vi "CRYOpen All.vi"   [LabVIEW 2013]
uses:
  CRYSystem/Typedef Control/CRYData Cluster.ctl
  CRYSystem/Typedef Control/CRYWaveform Cluster.ctl
  Global/CRYCurve Library Global.vi
panel:
  # "Open All Data(Curves, Values,Results, Waveforms)"
types:
  T1 = cluster{"pattern label":string, "pattern":string}
  T2 = cluster{"pattern label":string, "pattern":string}[]
  T3 = enum16{"Left Button", "Center Button", "Right Button", "Window Close"}
  T4 = enum16{"OK", "Yes", "YesNo", "YesNoCancel", "ReplaceAppend"}
  T5 = cluster{"Color":u32, "Interpolation":u8, "Point Style":u8, "Line Style":u8, "Point Color":u32, "Line Width":u8, "Bar Plot Style":u8, "Fill To":i16}
  T6 = typedef "CRYData Cluster.ctl" = cluster{"Name":string, "Curve":cluster{"x":dbl, "y":dbl, "z":dbl}[], "X data":u16, "Y data":u16, "Z data":u16, "X axis":u16, "Y axis":u16, "Z axis":u16, "X unit":string, "Y unit":string, "Z unit":string, "X dB ref":dbl, "Y dB ref":dbl, "Z dB ref":dbl, "single val":bool, "protected":bool, "display X":bool, "display Y":bool, "display Z":bool, "Test Info":string, "Step No.":i32, "Plot Settings":cluster{"Color":u32, "Interpolation":u8, "Point Style":u8, "Line Style":u8, "Point Color":u32, "Line Width":u8, "Bar Plot Style":u8, "Fill To":i16}, "AutoProtect":bool}
  T7 = typedef "CRYResult Cluster.ctl" = cluster{"Name":string, "Margin":dbl, "unit":string, "Verdict":bool, "Limit":string, "Max/Min":string, "protected":bool, "Step No.":i32, "Test Info":string, "AutoProtect":bool}
  T8 = typedef "CRYWaveform Cluster.ctl" = cluster{"Waveform":cluster{"X0":dbl, "dX":dbl, "Y":sgl[]}, "X data":u16, "Y data":u16, "Y axis":u16, "X unit":string, "Y unit":string, "Y dB ref":dbl, "display Y":bool, "display X":bool, "Overload?":bool, "Test Info":string, "Step No.":i32, "Name":string, "protected":bool, "Sqc history":string[], "Signal Channel ID":i32, "Plot Settings":cluster{"Color":u32, "Interpolation":u8, "Point Style":u8, "Line Style":u8, "Point Color":u32, "Line Width":u8, "Bar Plot Style":u8, "Fill To":i16}, "AutoProtect":bool}
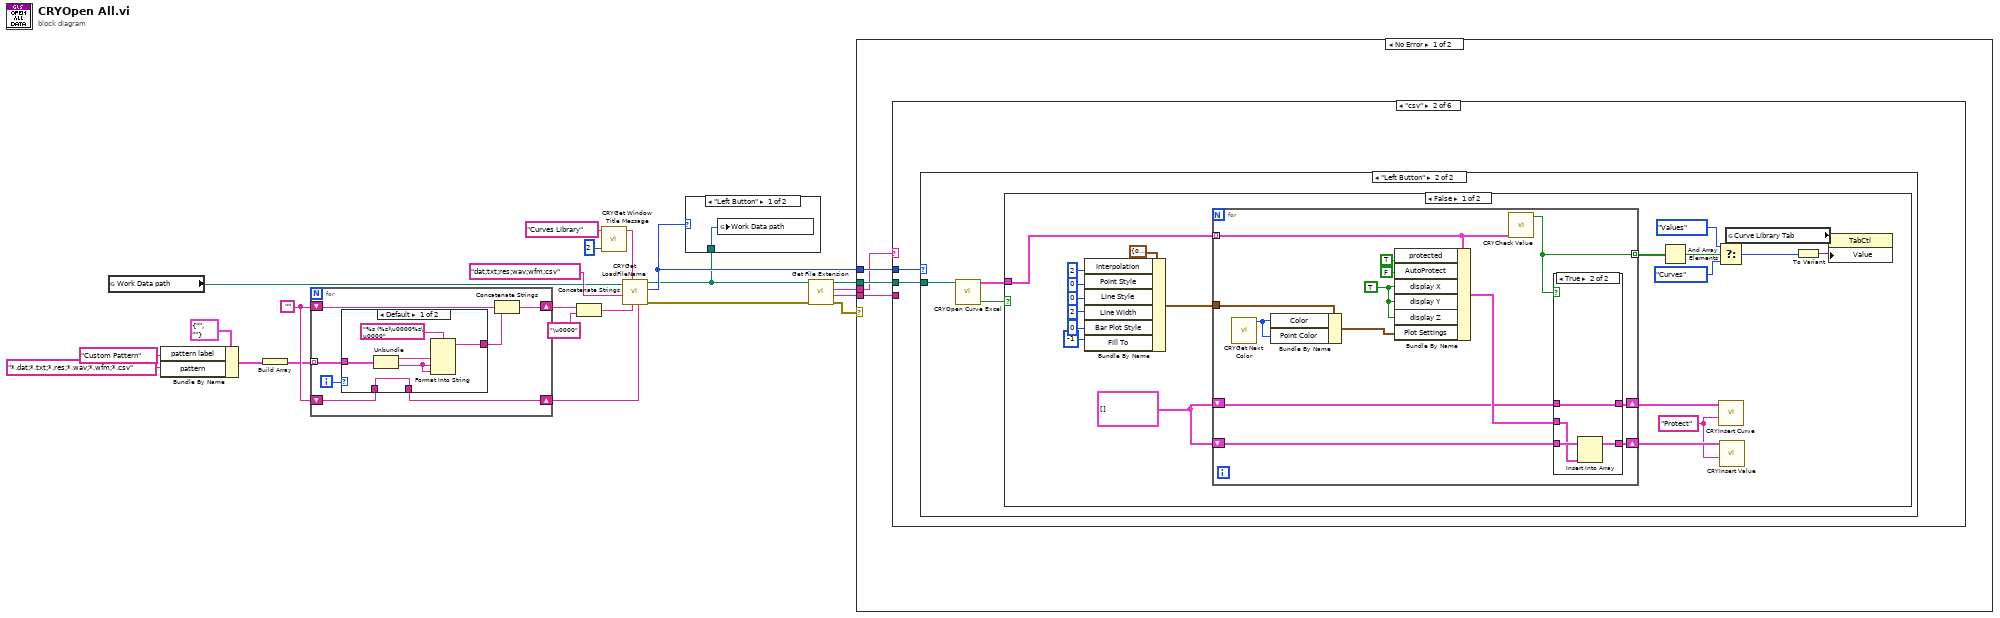
[diagram p0: block diagram]
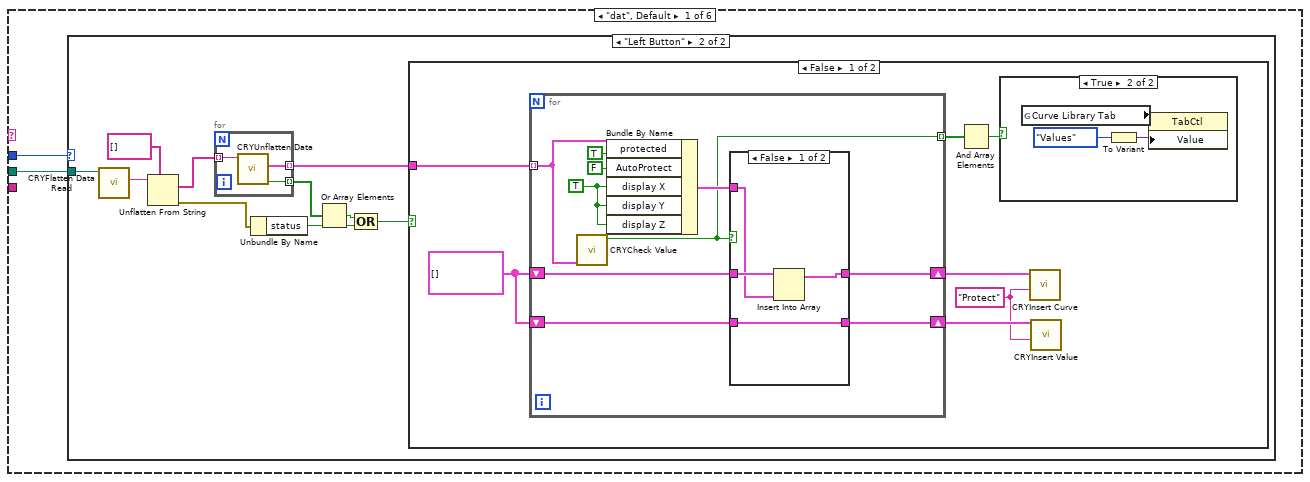
[diagram p3: hidden frame]
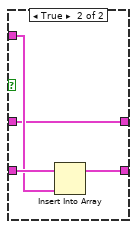
[diagram p6: hidden frame]
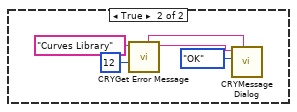
[diagram p7: hidden frame]
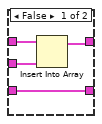
[diagram p9: hidden frame]
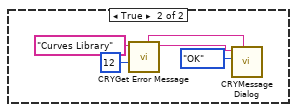
[diagram p10: hidden frame]
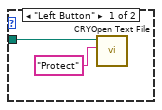
[diagram p12: hidden frame]
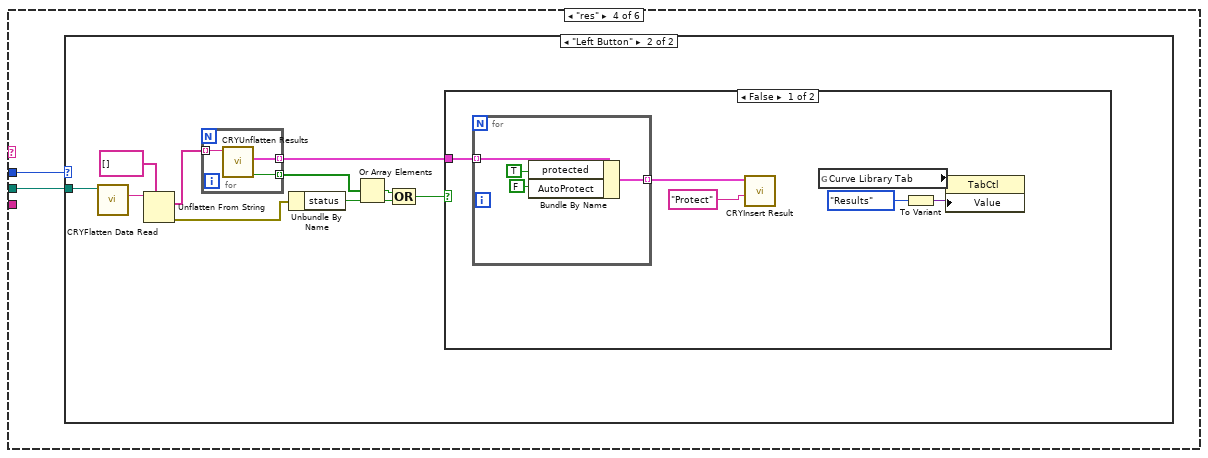
[diagram p13: hidden frame]
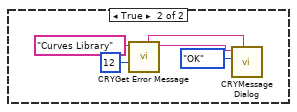
[diagram p15: hidden frame]
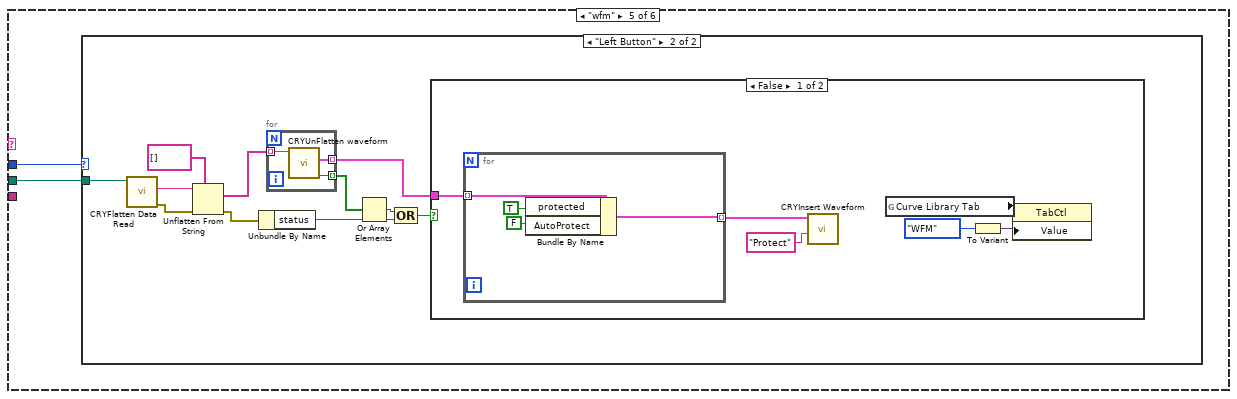
[diagram p16: hidden frame]
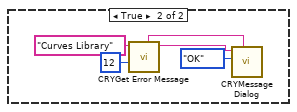
[diagram p18: hidden frame]
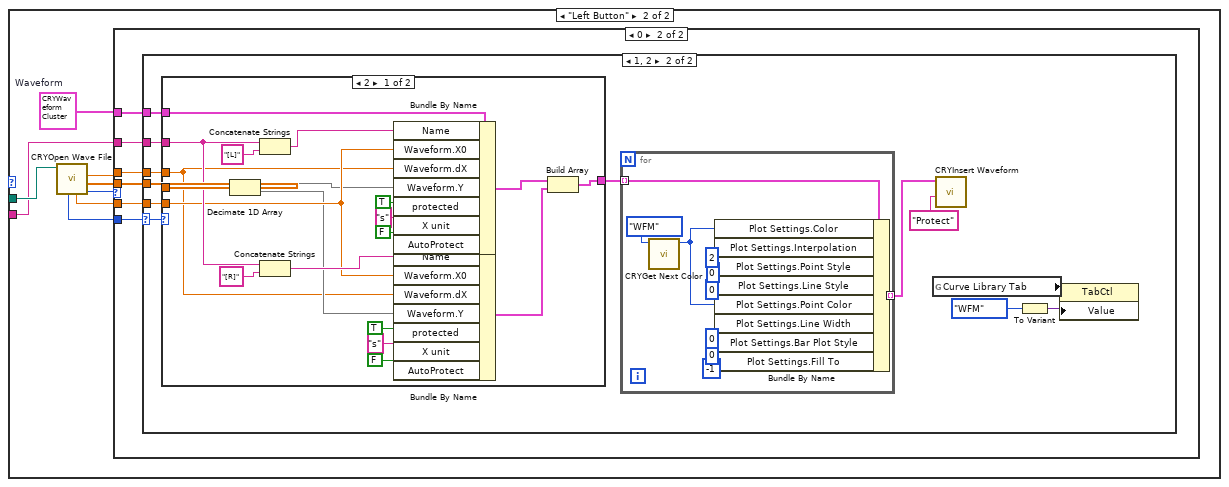
[diagram p20: hidden frame]
diagram:
  w14 = ""
  n1 = global read "CRYCurve Library Global.vi" "Work Data path"() -> (w3:path)
  n2 = Bundle By Name(cluster=T1 {"pattern label"="", "pattern"=""} ("File Types"), "pattern label"="Custom Pattern" ("pattern (all files)"), "pattern"="*.dat;*.txt;*.res;*.wav;*.wfm;*.csv" ("pattern (all files)")) -> (w5:T1)
  n3 = Build Array(w5) -> (w13:T2)
  n4 = for {
    tunnel: w13 -> [w29] mode=indexing
    shift-right: [w28] -> w16
    shift-left: w14 -> [w27]
    shift-right: [w24] -> w12
    shift-left: w14 -> [w23]
    i -> [w26]
    n5 = case shown="Default" w26 {
      tunnel: w29 -> [w35 w40]
      tunnel: [w31 w37] -> w25
      tunnel: [w30 w36] -> w24
      tunnel: w23 -> [w30 _]
      frame Default {
        n6 = Unbundle(w35) -> ("pattern label"=w34:string, "pattern"=w32:string)
        n7 = Format Into String(format string="%s (%s)\u0000%s\u0000", w34, w32, w32) -> (resulting string=w31:string)  [unwired: 2 in, 1 out]
      }
      frame 0 {
        n8 = Unbundle(w40) -> ("pattern label"=w36:string, "pattern"=w38:string)
        n9 = Format Into String(format string="%s)\u0000%s\u0000", w38, w38) -> (resulting string=w37:string)  [unwired: 2 in, 1 out]
      }
    }
    n10 = Concatenate Strings(w27, w25) -> (w28:string)
  }
  n11 = Concatenate Strings(w16, "\u0000" ("format string")) -> (w11:string)
  n12 = call "CRYGet Window Title Message.vi"("No"=2 ("Error No"), "Kind"="Curves Library") -> ("Multibyte String"=w17:string)  [unwired: 4 in, 5 out]
  n13 = call "CRYGet LoadFileName.vi"("pattern label"=w12, "pattern (all files)"=w11, "TitleName"=w17, "Category Name"="dat;txt;res;wav;wfm;csv" ("pattern (all files)"), "Start path"=w3) -> ("error out"=w21:errorcluster, "Which Button?"=w2:T3, "Path"=w1:path)  [unwired: 3 in, 1 out]
  n14 = case shown="\"Left Button\"" w2 {
    tunnel: w1 -> [w41 _]
    frame "Left Button" {
      n15 = global write "CRYCurve Library Global.vi" "Work Data path"(w41) -> ()
    }
    frame "Center Button", Default {
    }
  }
  n16 = call <vilib>:"Get File Extension.vi"("error in (no error)"=w21, "file"=w1) -> ("error out"=w9:errorcluster, "filename without extension"=w20:string, "lowercase file extension"=w19:string, "dup file"=w22:path)  [unwired: 6 out]
  n17 = case shown="No Error" w9 {
    tunnel: w2 -> [w45 _]
    tunnel: w22 -> [w44 _]
    tunnel: w20 -> [w43 _]
    tunnel: w19 -> [w42 _]
    frame No Error {
      n18 = case shown="\"csv\"" w42 {
        tunnel: w45 -> [w47 w95 w146 w150 w180 w212]
        tunnel: w44 -> [w46 w94 w145 w149 w179 w211]
        tunnel: w43 -> [_ _ _ _ _ w210]
        frame "dat", Default {
          n19 = case shown="\"Left Button\"" w47 {
            tunnel: w46 -> [_ w57]
            frame "Center Button", Default {
            }
            frame "Left Button" {
              n20 = call "CRYFlatten Data Read.vi"("Path In"=w57) -> ("Flatten Data Out"=w56:string)  [unwired: 1 in, 7 out]
              n21 = Unflatten From String(type=string[] [], binary string=w56) -> (value=w54:string[], error out=w50:errorcluster)  [unwired: 1 in, 3 out]
              n22 = for {
                tunnel: w54 -> [w60] mode=indexing
                tunnel: [w59] -> w53 mode=indexing
                tunnel: [w58] -> w48 mode=indexing
                n23 = call "CRYUnflatten Data.vi"("Unflatten data"=w60) -> ("Error?"=w58:bool, "Datum"=w59:T6)  [unwired: 8 in, 1 out]
              }
              n24 = Unbundle By Name(w50) -> ("status"=w51:bool)
              n25 = Or Array Elements(Boolean array=w48) -> (logical OR=w52:bool)
              n26 = Compound Arithmetic op=OR(w52, w51) -> (w49:bool)
              n27 = case shown="False" w49 {
                tunnel: w53 -> [w65 _]
                frame False {
                  w61 = "Protect" ("sOption")
                  w64 = T6[] []
                  n28 = for {
                    tunnel: w65 -> [w79] mode=indexing
                    tunnel: [w78] -> w67 mode=indexing
                    shift-right: [w71] -> w63
                    shift-left: w64 -> [w74]
                    shift-right: [w72] -> w62
                    shift-left: w64 -> [w73]
                    w75 = TRUE ("display X")
                    n29 = call "CRYCheck Value.vi"("Data"=w79) -> ("Single?"=w78:bool)  [unwired: 2 in, 8 out]
                    n30 = Bundle By Name(cluster=w79, "protected"=TRUE, "AutoProtect"=FALSE, "display X"=w75, "display Y"=w75, "display Z"=w75) -> (w80:T6)
                    n31 = case shown="False" w78 {
                      tunnel: w80 -> [w83 w87]
                      tunnel: w74 -> [w84 w85]
                      tunnel: w73 -> [w81 w88]
                      tunnel: [w81 w86] -> w72
                      tunnel: [w82 w85] -> w71
                      frame False {
                        n32 = Insert Into Array(array=w84, new element=w83) -> (w82:T6[])  [unwired: 1 in]
                      }
                      frame True {
                        n33 = Insert Into Array(array=w88, new element=w87) -> (w86:T6[])  [unwired: 1 in]
                      }
                    }
                  }
                  n34 = And Array Elements(Boolean array=w67) -> (logical AND=w66:bool)
                  n35 = case shown="True" w66 {
                    frame False {
                    }
                    frame True {
                      n36 = global read "CRYCurve Library Global.vi" "Curve Library Tab"() -> (w70:refnum<vi>)
                      n37 = To Variant(anything=enum32{"Curves", "Values", "Results", "WFM"}."Values" ("Value")) -> (Variant=w68:variant)
                      n38 = property class="TabCtl"(reference=w70, "Value"=w68) -> ()  [unwired: 1 in, 2 out]
                    }
                  }
                  n39 = call "CRYInsert Curve.vi"("sOption"=w61, "Curve"=w63) -> ()  [unwired: 2 in, 8 out]
                  n40 = call "CRYInsert Value.vi"("sOption"=w61, "Value"=w62) -> ()  [unwired: 2 in, 8 out]
                }
                frame True {
                  n41 = call "CRYGet Error Message.vi"("Error No"=12, "Kind"="Curves Library") -> ("Message"=w90:string, "Window Title"=w89:string)  [unwired: 4 in, 4 out]
                  n42 = call "CRYMessage Dialog.vi"("Window Title"=w89, "YesNoCancel"=T4."OK", "Message Content"=w90) -> ()  [unwired: 7 in, 2 out]
                }
              }
            }
          }
        }
        frame "csv" {
          n43 = case shown="\"Left Button\"" w95 {
            tunnel: w94 -> [_ w98]
            frame "Center Button", Default {
            }
            frame "Left Button" {
              n44 = call "CRYOpen Curve Excel .vi"("file path (dialog if empty)"=w98) -> ("Return"=w96:bool, "Data"=w97:T6[])  [unwired: 9 in]
              n45 = case shown="False" w96 {
                tunnel: w97 -> [w117 _]
                frame False {
                  w113 = "Protect" ("sOption")
                  w116 = T6[] []
                  n46 = Bundle By Name(cluster=T5 {"Color"=0, "Interpolation"=0, "Point Style"=0, "Line Style"=0, "Point Color"=0, "Line Width"=0, "Bar Plot Style"=0, "Fill To"=0} ("Plot Settings"), "Interpolation"=u8 2 ("Plot Settings.Interpolation"), "Point Style"=u8 0 ("Plot Settings.Point Style"), "Line Style"=u8 0 ("Plot Settings.Line Style"), "Line Width"=u8 2 ("Plot Settings.Line Width"), "Bar Plot Style"=u8 0 ("Plot Settings.Bar Plot Style"), "Fill To"=i16 -1 ("Plot Settings.Fill To")) -> (w99:T5)
                  n47 = for {
                    tunnel: w117 -> [w122] mode=indexing
                    tunnel: [w130] -> w118 mode=indexing
                    shift-right: [w123] -> w115
                    shift-left: w116 -> [w126]
                    shift-right: [w124] -> w114
                    shift-left: w116 -> [w125]
                    tunnel: w99 -> [w120]
                    w127 = TRUE ("display X")
                    n48 = call "CRYGet Next Color.vi"() -> ("Color"=w121:u32)  [unwired: 1 in, 10 out]
                    n49 = Bundle By Name(cluster=w120, "Color"=w121, "Point Color"=w121) -> (w119:T5)
                    n50 = Bundle By Name(cluster=w122, "protected"=TRUE, "AutoProtect"=FALSE, "display X"=w127, "display Y"=w127, "display Z"=w127, "Plot Settings"=w119) -> (w131:T6)
                    n51 = call "CRYCheck Value.vi"("Data"=w122) -> ("Single?"=w130:bool)  [unwired: 2 in, 8 out]
                    n52 = case shown="True" w130 {
                      tunnel: w131 -> [w134 w138]
                      tunnel: w126 -> [w135 w136]
                      tunnel: w125 -> [w132 w139]
                      tunnel: [w132 w137] -> w124
                      tunnel: [w133 w136] -> w123
                      frame False {
                        n53 = Insert Into Array(array=w135, new element=w134) -> (w133:T6[])  [unwired: 1 in]
                      }
                      frame True {
                        n54 = Insert Into Array(array=w139, new element=w138) -> (w137:T6[])  [unwired: 1 in]
                      }
                    }
                  }
                  n55 = And Array Elements(Boolean array=w118) -> (logical AND=w110:bool)
                  n56 = Select(t=enum32{"Curves", "Values", "Results", "WFM"}."Values" ("Value"), s=w110, f=enum32{"Curves", "Values", "Results", "WFM"}."Curves" ("Value")) -> (s? t:f=w107:enum32{"Curves", "Values", "Results", "WFM"})
                  n57 = call "CRYInsert Curve.vi"("sOption"=w113, "Curve"=w115) -> ()  [unwired: 2 in, 8 out]
                  n58 = call "CRYInsert Value.vi"("sOption"=w113, "Value"=w114) -> ()  [unwired: 2 in, 8 out]
                  n59 = global read "CRYCurve Library Global.vi" "Curve Library Tab"() -> (w112:refnum<vi>)
                  n60 = To Variant(anything=w107) -> (Variant=w111:variant)
                  n61 = property class="TabCtl"(reference=w112, "Value"=w111) -> ()  [unwired: 1 in, 2 out]
                }
                frame True {
                  n62 = call "CRYGet Error Message.vi"("Error No"=12, "Kind"="Curves Library") -> ("Message"=w141:string, "Window Title"=w140:string)  [unwired: 4 in, 4 out]
                  n63 = call "CRYMessage Dialog.vi"("Window Title"=w140, "YesNoCancel"=T4."OK", "Message Content"=w141) -> ()  [unwired: 7 in, 2 out]
                }
              }
            }
          }
        }
        frame "txt" {
          n64 = case shown="\"Center Button\", Default" w146 {
            tunnel: w145 -> [w148 _]
            frame "Left Button" {
              n65 = call "CRYOpen Text File.vi"("sOption"="Protect", "File Path"=w148) -> ()  [unwired: 8 in, 2 out]
            }
            frame "Center Button", Default {
            }
          }
        }
        frame "res" {
          n66 = case shown="\"Left Button\"" w150 {
            tunnel: w149 -> [_ w160]
            frame "Center Button", Default {
            }
            frame "Left Button" {
              n67 = call "CRYFlatten Data Read.vi"("Path In"=w160) -> ("Flatten Data Out"=w159:string)  [unwired: 1 in, 7 out]
              n68 = Unflatten From String(type=string[] [], binary string=w159) -> (value=w157:string[], error out=w152:errorcluster)  [unwired: 2 in, 2 out]
              n69 = for {
                tunnel: w157 -> [w163] mode=indexing
                tunnel: [w162] -> w156 mode=indexing
                tunnel: [w161] -> w153 mode=indexing
                n70 = call "CRYUnflatten Results.vi"("Unflatten Result"=w163) -> ("Error?"=w161:bool, "Result"=w162:T7)  [unwired: 8 in, 1 out]
              }
              n71 = Unbundle By Name(w152) -> ("status"=w154:bool)
              n72 = Or Array Elements(Boolean array=w153) -> (logical OR=w155:bool)
              n73 = Compound Arithmetic op=OR(w155, w154) -> (w151:bool)
              n74 = case shown="False" w151 {
                tunnel: w156 -> [w169 _]
                frame False {
                  n75 = for {
                    tunnel: w169 -> [w173] mode=indexing
                    tunnel: [w170] -> w168 mode=indexing
                    n76 = Bundle By Name(cluster=w173, "protected"=TRUE, "AutoProtect"=FALSE) -> (w170:T7)
                  }
                  n77 = call "CRYInsert Result.vi"("sOption"="Protect", "Result"=w168) -> ()  [unwired: 2 in, 8 out]
                  n78 = global read "CRYCurve Library Global.vi" "Curve Library Tab"() -> (w166:refnum<vi>)
                  n79 = To Variant(anything=enum32{"Curves", "Values", "Results", "WFM"}."Results" ("Value")) -> (Variant=w164:variant)
                  n80 = property class="TabCtl"(reference=w166, "Value"=w164) -> ()  [unwired: 1 in, 2 out]
                }
                frame True {
                  n81 = call "CRYGet Error Message.vi"("Error No"=12, "Kind"="Curves Library") -> ("Message"=w175:string, "Window Title"=w174:string)  [unwired: 4 in, 4 out]
                  n82 = call "CRYMessage Dialog.vi"("Window Title"=w174, "YesNoCancel"=T4."OK", "Message Content"=w175) -> ()  [unwired: 7 in, 2 out]
                }
              }
            }
          }
        }
        frame "wfm" {
          n83 = case shown="\"Left Button\"" w180 {
            tunnel: w179 -> [_ w191]
            frame "Center Button", Default {
            }
            frame "Left Button" {
              n84 = call "CRYFlatten Data Read.vi"("Path In"=w191) -> ("error out"=w189:errorcluster, "Flatten Data Out"=w190:string)  [unwired: 1 in, 6 out]
              n85 = Unflatten From String(type=string[] [], binary string=w190, error in (no error)=w189) -> (value=w187:string[], error out=w185:errorcluster)  [unwired: 3 out]
              n86 = Unbundle By Name(w185) -> ("status"=w182:bool)
              n87 = for {
                tunnel: w187 -> [w194] mode=indexing
                tunnel: [w193] -> w186 mode=indexing
                tunnel: [w192] -> w184 mode=indexing
                n88 = call "CRYUnFlatten waveform.vi"("Unflatten Waveform"=w194) -> ("Error?"=w192:bool, "Waveform Cluster"=w193:T8)  [unwired: 8 in, 1 out]
              }
              n89 = Or Array Elements(Boolean array=w184) -> (logical OR=w183:bool)
              n90 = Compound Arithmetic op=OR(w183, w182) -> (w181:bool)
              n91 = case shown="False" w181 {
                tunnel: w186 -> [w200 _]
                frame False {
                  n92 = for {
                    tunnel: w200 -> [w204] mode=indexing
                    tunnel: [w201] -> w198 mode=indexing
                    n93 = Bundle By Name(cluster=w204, "protected"=TRUE, "AutoProtect"=FALSE) -> (w201:T8)
                  }
                  n94 = call "CRYInsert Waveform.vi"("sOption"="Protect", "Waveform"=w198) -> ()  [unwired: 2 in, 8 out]
                  n95 = global read "CRYCurve Library Global.vi" "Curve Library Tab"() -> (w197:refnum<vi>)
                  n96 = To Variant(anything=enum32{"Curves", "Values", "Results", "WFM"}."WFM" ("Value")) -> (Variant=w195:variant)
                  n97 = property class="TabCtl"(reference=w197, "Value"=w195) -> ()  [unwired: 1 in, 2 out]
                }
                frame True {
                  n98 = call "CRYGet Error Message.vi"("Error No"=12, "Kind"="Curves Library") -> ("Message"=w206:string, "Window Title"=w205:string)  [unwired: 4 in, 4 out]
                  n99 = call "CRYMessage Dialog.vi"("Window Title"=w205, "YesNoCancel"=T4."OK", "Message Content"=w206) -> ()  [unwired: 7 in, 2 out]
                }
              }
            }
          }
        }
        frame "wav" {
          n100 = case shown="\"Center Button\", Default" w212 {
            tunnel: w211 -> [_ w220]
            tunnel: w210 -> [_ w214]
            frame "Center Button", Default {
            }
            frame "Left Button" {
              w213 = T8 {"Waveform"={"X0"=0.0, "dX"=0.0, "Y"=[]}, "X data"=1, "Y data"=1, "Y axis"=1, "X unit"="s", "Y unit"="V", "Y dB ref"=1.0, "display Y"=TRUE, "display X"=TRUE, "Overload?"=FALSE, "Test Info"="", "Step No."=0, "Name"="", "protected"=FALSE, "Sqc history"=[], "Signal Channel ID"=0, "Plot Settings"={"Color"=0, "Interpolation"=0, "Point Style"=0, "Line Style"=0, "Point Color"=0, "Line Width"=0, "Bar Plot Style"=0, "Fill To"=0}, "AutoProtect"=FALSE}  # Waveform
              n101 = call "CRYOpen Wave File.vi"("Wave File Path In"=w220) -> ("Error Out(0-OK)"=w219:u32, "Wave Data Out"=w216:sgl[], "dT"=w217:dbl, "X0"=w218:dbl, "Channels"=w215:u32)  [unwired: 5 in, 1 out]
              n102 = case shown="0" w219 {
                tunnel: w213 -> [_ w231]
                tunnel: w218 -> [_ w230]
                tunnel: w217 -> [_ w229]
                tunnel: w216 -> [_ w228]
                tunnel: w215 -> [_ w227]
                tunnel: w214 -> [_ w226]
                frame Default {
                  n103 = call "CRYGet Error Message.vi"("Error No"=7, "Kind"="Curves Library") -> ("Message"=w221:string, "Window Title"=w222:string)  [unwired: 4 in, 4 out]
                  n104 = call "CRYMessage Dialog.vi"("Window Title"=w222, "YesNoCancel"=T4."OK", "Message Content"=w221) -> ()  [unwired: 7 in, 2 out]
                }
                frame 0 {
                  n105 = case shown="1, 2" w227 {
                    selector: w227 -> [_ w244]
                    tunnel: w231 -> [_ w248]
                    tunnel: w230 -> [_ w247]
                    tunnel: w229 -> [_ w246]
                    tunnel: w228 -> [_ w245]
                    tunnel: w226 -> [_ w242]
                    frame 0, Default {
                      n106 = call "CRYGet Error Message.vi"("Error No"=6, "Kind"="Curves Library") -> ("Message"=w232:string, "Window Title"=w233:string)  [unwired: 4 in, 4 out]
                      n107 = call "CRYMessage Dialog.vi"("Window Title"=w233, "YesNoCancel"=T4."OK", "Message Content"=w232) -> ()  [unwired: 7 in, 2 out]
                    }
                    frame 1, 2 {
                      n108 = case shown="2" w244 {
                        tunnel: w248 -> [w269 w288]
                        tunnel: w242 -> [w268 w284]
                        tunnel: w247 -> [w267 w283]
                        tunnel: w246 -> [w264 w282]
                        tunnel: w245 -> [w276 w281]
                        tunnel: [w261 w280] -> w241
                        frame 2 {
                          n109 = Decimate 1D Array(w276) -> (w266:sgl[], w265:sgl[])
                          n110 = Concatenate Strings(w268, "[L]" ("string")) -> (w274:string)
                          n111 = Concatenate Strings(w268, "[R]" ("string")) -> (w273:string)
                          n112 = Bundle By Name(cluster=w269, "Name"=w274, "Waveform.X0"=w267, "Waveform.dX"=w264, "Waveform.Y"=w266, "protected"=TRUE, "X unit"="s", "AutoProtect"=FALSE) -> (w263:T8)
                          n113 = Bundle By Name(cluster=w269, "Name"=w273, "Waveform.X0"=w267, "Waveform.dX"=w264, "Waveform.Y"=w265, "protected"=TRUE, "X unit"="s", "AutoProtect"=FALSE) -> (w262:T8)
                          n114 = Build Array(w263, w262) -> (w261:T8[])
                        }
                        frame 1, Default {
                          n115 = Bundle By Name(cluster=w288, "Name"=w284, "Waveform.X0"=w283, "Waveform.dX"=w282, "Waveform.Y"=w281, "protected"=TRUE, "X unit"="s", "AutoProtect"=FALSE) -> (w286:T8)
                          n116 = Build Array(w286) -> (w280:T8[])
                        }
                      }
                      n117 = for {
                        tunnel: w241 -> [w250] mode=indexing
                        tunnel: [w249] -> w240 mode=indexing
                        n118 = call "CRYGet Next Color.vi"("Type"=enum16{"Curves", "Values", "Results", "WFM"}."WFM") -> ("Color"=w254:u32)  [unwired: 10 out]
                        n119 = Bundle By Name(cluster=w250, "Plot Settings.Color"=w254, "Plot Settings.Interpolation"=u8 2, "Plot Settings.Point Style"=u8 0, "Plot Settings.Line Style"=u8 0, "Plot Settings.Point Color"=w254, "Plot Settings.Line Width"=u8 0, "Plot Settings.Bar Plot Style"=u8 0, "Plot Settings.Fill To"=i16 -1) -> (w249:T8)
                      }
                      n120 = global read "CRYCurve Library Global.vi" "Curve Library Tab"() -> (w239:refnum<vi>)
                      n121 = call "CRYInsert Waveform.vi"("sOption"="Protect", "Waveform"=w240) -> ()  [unwired: 2 in, 8 out]
                      n122 = To Variant(anything=enum32{"Curves", "Values", "Results", "WFM"}."WFM" ("Value")) -> (Variant=w237:variant)
                      n123 = property class="TabCtl"(reference=w239, "Value"=w237) -> ()  [unwired: 1 in, 2 out]
                    }
                  }
                }
              }
            }
          }
        }
      }
    }
    frame Error {
    }
  }
